vi "CrashScreen (SubVI).vi"(8 "error in (no error)":errorcluster, 11 "Display Queue in":refnum<queue>) -> (0 "error out":errorcluster, 3 "Display Queue out":refnum<queue>)   [LabVIEW 2017]
uses:
  Controls/DisplayControl.ctl
  Controls/DisplayCommand.ctl
  Controls/UpdateMessageControl.ctl
  Controls/UpdateMessageCommand.ctl
  Controls/UpdateMenuCommand.ctl
  Controls/EnableDisableCommand.ctl
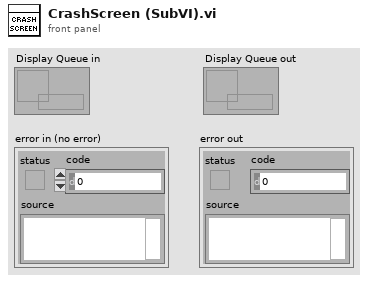
[diagram p1: front panel]
types:
  T1 = typedef "DisplayControl.ctl" = cluster{"Command":T2, "Data":variant}
  T2 = typedef "DisplayCommand.ctl" = enum16{"Initialize", "Open/Close Parcel", "Enable/Disable Controls", "FocusCursor", "UpdateMessage", "UpdateMenus", "FinishOperation", "Exit", "CleanUserInput"}
  T3 = typedef "EnableDisableCommand.ctl" = enum16{"InitialSetup", "StartOperation", "EnableUserInput", "DisableUserInput", "EnableMenus", "DisableMenus"}
  T4 = typedef "UpdateMenuCommand.ctl" = enum16{"MainMenu", "NoMenu"}
  T5 = typedef "UpdateMessageControl.ctl" = cluster{"Command":T6, "Data":variant}
  T6 = typedef "UpdateMessageCommand.ctl" = enum16{"SystemCrash2", "SystemCrash1", "Welcome", "MainMenu", "PhoneNumberFailed", "PhoneNumberSuccess", "ParcelNumberSuccess", "ParcelNumbertFailed", "SessionTerminate", "SessionFinished", "Deposit", "DepositComplete", "Withdrawal", "WithdrawalComplete", "WithdrawalFailed"}
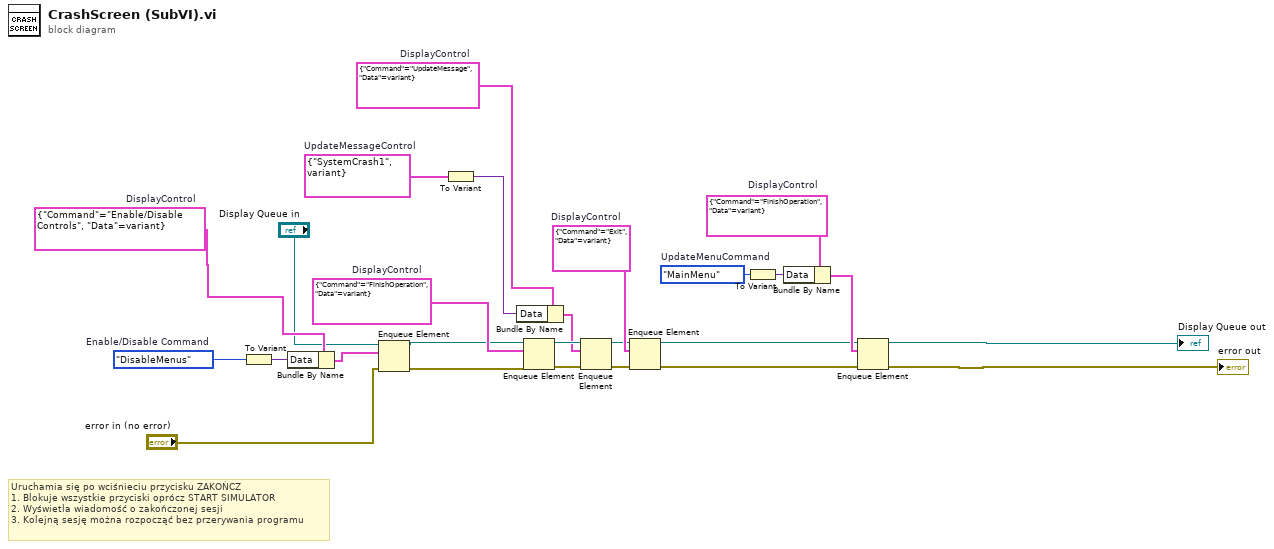
[diagram p0: block diagram]
diagram:
  w7 = T1 {"Command"=enum."Enable/Disable Controls", "Data"=variant}  # DisplayControl
  w9 = EnableDisableCommand."DisableMenus"  # Enable/Disable Command
  w11 = T1 {"Command"=enum."FinishOperation", "Data"=variant}  # DisplayControl
  w16 = T1 {"Command"=enum."FinishOperation", "Data"=variant}  # DisplayControl
  w17 = UpdateMenuCommand."MainMenu"  # UpdateMenuCommand
  w19 = T5 {"Command"=enum."SystemCrash1", "Data"=variant}  # UpdateMessageControl
  w21 = T1 {"Command"=enum."UpdateMessage", "Data"=variant}  # DisplayControl
  w26 = T1 {"Command"=enum."Exit", "Data"=variant}  # DisplayControl
  # "Uruchamia się po wciśnieciu przycisku ZAKOŃCZ\n1. Blokuje wszystkie przyciski oprócz START SIMULATOR\n2. Wyświetla wiadomość o zakończonej sesji\n3. Kolejną sesję można rozpocząć bez przerywania programu"
  n1 = To Variant(anything=w9) -> (Variant=w10:variant)
  n2 = Bundle By Name(cluster=w7, "Data"=w10) -> (w8:T1)
  n3 = Enqueue Element(queue="Display Queue in", element=w8, error in (no error)="error in (no error)") -> (queue out=w5:refnum<queue>, error out=w3:errorcluster)  [unwired: 1 in, 1 out]
  n4 = To Variant(anything=w19) -> (Variant=w20:variant)
  n5 = Bundle By Name(cluster=w21, "Data"=w20) -> (w18:T1)
  n6 = Enqueue Element(queue=w5, element=w11, error in (no error)=w3) -> (queue out=w24:refnum<queue>, error out=w23:errorcluster)  [unwired: 1 in, 1 out]
  n7 = Enqueue Element(queue=w24, element=w18, error in (no error)=w23) -> (queue out=w22:refnum<queue>, error out=w25:errorcluster)  [unwired: 1 in, 1 out]
  n8 = Enqueue Element(queue=w22, element=w26, error in (no error)=w25) -> (queue out=w13:refnum<queue>, error out=w12:errorcluster)  [unwired: 1 in, 1 out]
  n9 = To Variant(anything=w17) -> (Variant=w14:variant)
  n10 = Bundle By Name(cluster=w16, "Data"=w14) -> (w15:T1)
  n11 = Enqueue Element(queue=w13, element=w15, error in (no error)=w12) -> (queue out=→"Display Queue out":refnum<queue>, error out=→"error out":errorcluster)  [unwired: 1 in, 1 out]
